vi "Forward by Actor.vi"(6 "Message Priority (Normal)":T1=enum."Normal", 7 "Target Actor index(-1, all)":i32=-1, 8 "error in (no error)":errorcluster, 9 "Message":refnum<class "Message.lvclass">, 10 "Target Actor":refnum<class "Actor.lvclass">, 11 "Publisher in":refnum<class "Publisher.lvclass">) -> (0 "error out":errorcluster, 1 "Message forwarded?":bool, 3 "Publisher out":refnum<class "Publisher.lvclass">)   [LabVIEW 2020, in "Publisher.lvlib" / "Publisher.lvclass"]
doc: "Send 'Message' to actor(s) with 'Target Actor base name'. As default all actors with the name are addressed. A single specific actor can be specified using 'Target Actor index'."
uses:
  Publisher.lvclass
  PPL/HDH.Actor Framework.Core.Actor.lvlibp/1abvi3w/vi.lib/ActorFramework/Message Enqueuer/Message Priority.ctl
  PPL/HDH.Actor Framework.Core.Actor.lvlibp/1abvi3w/vi.lib/ActorFramework/Message/Message.lvclass
  PPL/HDH.Actor Framework.Core.Actor.lvlibp/1abvi3w/vi.lib/ActorFramework/Actor/Actor.lvclass
  Publisher.lvclass/Publisher.ctl
  1879999a-615c-413f-9ac1-690b47381e01.vi
  PPL/HDH.Actor Framework.Core.Actor.lvlibp/1abvi3w/vi.lib/ActorFramework/Message Enqueuer/Message Enqueuer.lvclass
  PPL/HDH.Actor Framework.Core.Utility.lvlibp
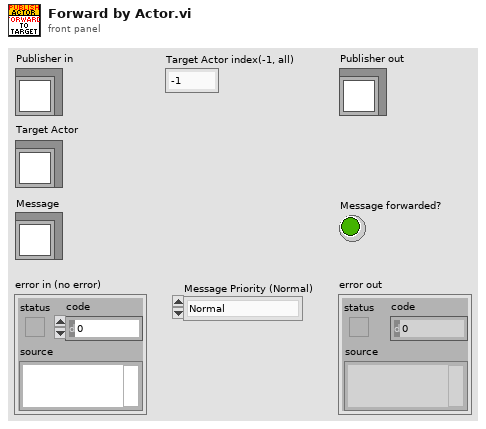
[diagram p1: front panel]
types:
  T1 = typedef "HDH.Actor Framework.Core.Actor.lvlibp/Message Enqueuer.lvclass/Message Priority.ctl" = enum16{"Low", "Normal", "High"}
  T2 = typedef "Publisher.lvlib/Publisher.lvclass/Ctl_Subscription Element.ctl" = cluster{"Object":refnum<class>, "Enqueuers":refnum<class "Message Enqueuer.lvclass">[]}
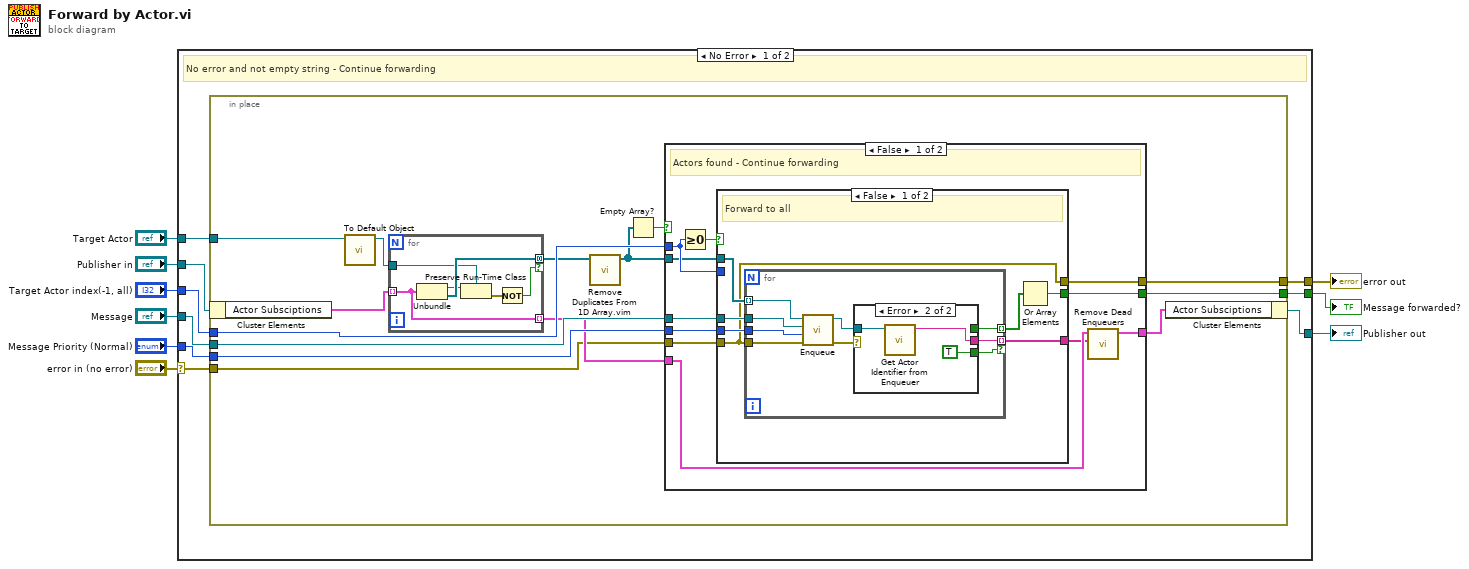
[diagram p0: block diagram]
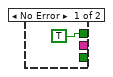
[diagram p2: hidden frame]
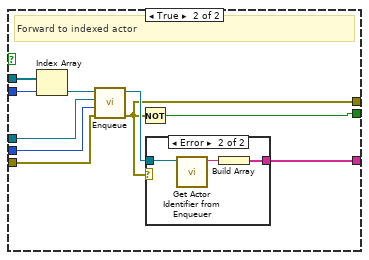
[diagram p3: hidden frame]
diagram:
  n1 = case shown="No Error" "error in (no error)" {
    selector: "error in (no error)" -> [w10 w85]
    tunnel: [w15 w85] -> w9
    tunnel: [w14 w86] -> w7
    tunnel: "Publisher in" -> [w18 w86]
    tunnel: [w16 _] -> w6
    tunnel: "Target Actor" -> [w17 _]
    tunnel: "Target Actor index(-1, all)" -> [w13 _]
    tunnel: "Message" -> [w12 _]
    tunnel: "Message Priority (Normal)" -> [w11 _]
    frame No Error {
      # "No error and not empty string - Continue forwarding"
      n2 = in-place {
        in-place-border: w17 -> [w27]
        in-place-border: w10 -> [w21]
        in-place-border: [w32] -> w16
        in-place-border: [w31] -> w15
        in-place-border: w13 -> [w30]
        in-place-border: w12 -> [w29]
        in-place-border: w11 -> [w28]
        n3 = in-place-cluster #1(w18) -> ("Actor Subsciptions"=w26:T2[])
        n4 = call "To Default Object.vi"("Object in"=w27) -> ("Default out"=w25:refnum<class "Actor.lvclass">)  [unwired: 10 in]
        n5 = for {
          tunnel: w25 -> [w33]
          tunnel: w26 -> [w35] mode=indexing
          tunnel: [w37] -> w24 mode=concatenating if=w36
          tunnel: [w35] -> w22 mode=indexing
          n6 = Unbundle(w35) -> ("Object"=w34:refnum<class>, "Enqueuers"=w37:refnum<class "Message Enqueuer.lvclass">[])
          n7 = Preserve Run-Time Class(object in=w34, 2:w33) -> (error out=w38:errorcluster)  [unwired: 1 in, 1 out]
          n8 = Not(x=w38) -> (.not. x?=w36:bool)
        }
        n9 = call "Remove Duplicates From 1D Array.vim"("array"=w24) -> ("array with duplicates removed"=w20:refnum<class "Message Enqueuer.lvclass">[])  [unwired: 10 in]
        n10 = Empty Array?(array=w20) -> (empty?=w19:bool)
        n11 = case shown="False" w19 {
          tunnel: [w44 _] -> w32
          tunnel: [w45 w83] -> w31
          tunnel: w30 -> [w48 _]
          tunnel: w29 -> [w47 _]
          tunnel: w28 -> [w46 _]
          tunnel: [w42 w84] -> w23
          tunnel: w22 -> [w43 w84]
          tunnel: w20 -> [w41 _]
          tunnel: w21 -> [w39 w83]
          frame False {
            # "Actors found - Continue forwarding"
            n12 = Greater Or Equal To 0?(x=w48) -> (x >= 0?=w49:bool)
            n13 = case shown="False" w49 {
              tunnel: w48 -> [_ w77]
              tunnel: w47 -> [w56 w79]
              tunnel: w46 -> [w55 w78]
              tunnel: [w50 w70] -> w45
              tunnel: [w54 w72] -> w44
              tunnel: w41 -> [w53 w76]
              tunnel: [w52 w73] -> w40
              tunnel: w39 -> [w50 w71]
              frame False {
                # "Forward to all"
                n14 = for {
                  tunnel: w56 -> [w65]
                  tunnel: w55 -> [w64]
                  tunnel: w53 -> [w63] mode=indexing
                  tunnel: [w60] -> w52 mode=indexing if=w59
                  tunnel: [w58] -> w51 mode=indexing
                  tunnel: w50 -> [w57]
                  n15 = call "Enqueue.vi"("error in (no error)"=w57, "Message Priority (Normal)"=w64, "Message"=w65, "Message Enqueuer in"=w63) -> ("error out"=w61:errorcluster, "Message Enqueuer out"=w62:refnum<class "Message Enqueuer.lvclass">)  [unwired: 6 in]
                  n16 = case shown="Error" w61 {
                    tunnel: w62 -> [_ w69]
                    tunnel: [_ w68] -> w60
                    tunnel: [_ TRUE] -> w59
                    tunnel: [TRUE _] -> w58
                    frame No Error {
                    }
                    frame Error {
                      n17 = call "Get Actor Identifier from Enqueuer.vi"("Message Enqueuer in"=w69) -> ("Actor ID string out"=w68:string)  [unwired: 9 in, 1 out]
                    }
                  }
                }
                n18 = Or Array Elements(Boolean array=w51) -> (logical OR=w54:bool)
              }
              frame True {
                # "Forward to indexed actor"
                n19 = Index Array(array=w76, index=w77) -> (element=w75:refnum<class "Message Enqueuer.lvclass">)
                n20 = call "Enqueue.vi"("error in (no error)"=w71, "Message Priority (Normal)"=w78, "Message"=w79, "Message Enqueuer in"=w75) -> ("error out"=w70:errorcluster, "Message Enqueuer out"=w74:refnum<class "Message Enqueuer.lvclass">)  [unwired: 6 in]
                n21 = Not(x=w70) -> (.not. x?=w72:bool)
                n22 = case shown="Error" w70 {
                  tunnel: w74 -> [_ w82]
                  tunnel: [_ w80] -> w73
                  frame No Error {
                  }
                  frame Error {
                    n23 = call "Get Actor Identifier from Enqueuer.vi"("Message Enqueuer in"=w82) -> ("Actor ID string out"=w81:string)  [unwired: 9 in, 1 out]
                    n24 = Build Array(w81) -> (w80:string[])
                  }
                }
              }
            }
            n25 = call "Remove Dead Enqueuers.vi"("Enqueuers to remove"=w40, "Subsciptions in"=w43) -> ("Subsciptions out"=w42:T2[])  [unwired: 8 in, 1 out]
          }
          frame True {
            # "No actors found - Abort operation"
          }
        }
        n26 = in-place-cluster #1("Actor Subsciptions"=w23) -> (w14:refnum<class "Publisher.lvclass">)
      }
    }
    frame Error {
      # "Error or no target - Abort operation"
    }
  }
  "error out" <- w9
  "Publisher out" <- w7
  "Message forwarded?" <- w6
